vi "Package.vi"   [LabVIEW 2017, in "Scripts.lvlib"]
doc: "Builds a VI package (vip) for this project for LabVIEW 2015."
uses:
  Scripts.lvlib
  Controls/LabVIEW Versions.ctl
panel:
  # "Overview: Builds a VI Package (vip) for LabVIEW versions >= 2015\nRequirements: LabVIEW 2015, VIPM Pro, VIPM API\nInstructions: Run this VI.\n\nThis VI attempts automate the building the VIP file for this add-on as much as possible. If VIPM Pro is not available, then the VIPM API will not work, and the building of the package must be done manually. This VI automates the following manual steps:\n\n1. Save the current project for LabVIEW 2015\n    a. From the Project Explorer window, select File>>Save for Previous Version... A new dialog will appear.\n    b. Select 15.0 from the drop down menu.\n    c. Click Save.... A new dialog will appear. Create a \"target\\15.0\" folder hierarchy in the root project folder (same location as the project file,    \n        .lvproj) if it does not already exist.\n    d. Click OK. All of the contents of the project will be saved to LabVIEW 2015.\n2. Copy the Help source to the target output\n    a. Start Windows Explorer.\n    b. Navigate to the \"<project root>\\src\" folder in Windows Explorer.\n    c. Copy the \"Help\" folder to the \"target\\15.0\\src\" location.\n3. Start LabVIEW 2015 and open the \"target\\15.0\\Alphabetize Cluster Elements.lvproj\" file created in Step 1. Do NOT open any file in the \"target\\15.0\" folder in any other \n    version of LabVIEW.\n4. Build all Source Distributions defined under \"Build Specifications\" tree item in the Project Explorer. A new \"target\\15.0\\builds\" folder will be \n    created with a sub-folder for each component.\n5. Expand the \"Configs\" virtual folder in the Project Explorer and double click on the \"Alphabetize Cluster Elements.vipb\" file. This will start the VIPM application.\n6. Click the \"Build\" icon near the top of the window for the Eulogy package specification. Do NOT alter any values, but ensure \"2015\" is selected at \n    the top right.\n7. Once the package is built, it will be available at \"target\\15.0\\packages\". \n\nNote, any version newer than LabVIEW 2015 can be used to run this VI and still have the package built for LabVIEW 2015, but the LabVIEW 2015 development environment must be installed.\n\nWhen this VI runs, it will automatically start LabVIEW 2015, build all of the components, start VIPM, build the package, then close both LabVIEW 2015 and VIPM. Another VI, \"Build Target.vi\" will run during this process. Do not abort or close the VI will running.\n\nThe oldest LabVIEW version possible for this add-on is LabVIEW 2015. LabVIEW 2015 introduced shortcut menu plugins, which are an integral usability component to this add-on. If the shortcut menu items are not needed, then the oldest version possible is LabVIEW 2013, which introduced custom bookmark managers. Similarly, custom bookmark managers are an integratl usability component for this add-on. All of the features and functionality are not possible with versions older than LabVIEW 2015."
types:
  T1 = typedef "Scripts.lvlib/LabVIEW Versions.ctl" = enum16{"2009", "2010", "2011", "2012", "2013", "2014", "2015", "2016", "2017", "2018"}
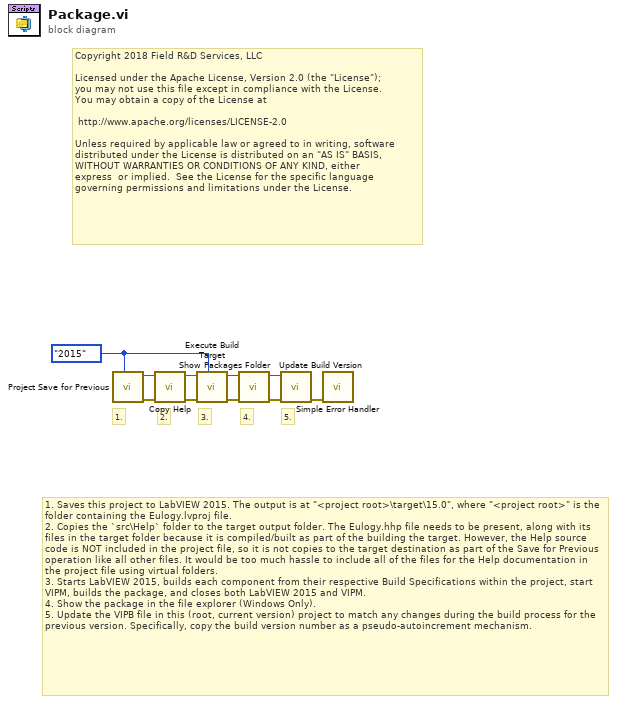
[diagram p0: block diagram]
diagram:
  w10 = LabVIEW_Versions."2015" ("LabVIEW Previous Version")
  # "5."
  # "4."
  # "3."
  # "2."
  # "Copyright 2018 Field R&D Services, LLC\n\nLicensed under the Apache License, Version 2.0 (the \"License\");\nyou may not use this file except in compliance with the License.\nYou may obtain a copy of the License at\n\n\thttp://www.apache.org/licenses/LICENSE-2.0\n\nUnless required by applicable law or agreed to in writing, software\ndistributed under the License is distributed on an \"AS IS\" BASIS,\nWITHOUT WARRANTIES OR CONDITIONS OF ANY KIND, either \nexpress  or implied.  See the License for the specific language \ngoverning permissions and limitations under the License."
  # "1. Saves this project to LabVIEW 2015. The output is at \"<project root>\\target\\15.0\", where \"<project root>\" is the folder containing the Eulogy.lvproj file.\n2. Copies the `src\\Help` folder to the target output folder. The Eulogy.hhp file needs to be present, along with its files in the target folder because it is compiled/built as part of the building the target. However, the Help source code is NOT included in the project file, so it is not copies to the target destination as part of the Save for Previous operation like all other files. It would be too much hassle to include all of the files for the Help documentation in the project file using virtual folders.\n3. Starts LabVIEW 2015, builds each component from their respective Build Specifications within the project, start VIPM, builds the package, and closes both LabVIEW 2015 and VIPM.\n4. Show the package in the file explorer (Windows Only).\n5. Update the VIPB file in this (root, current version) project to match any changes during the build process for the previous version. Specifically, copy the build version number as a pseudo-autoincrement mechanism."
  # "1."
  n1 = call "Project Save for Previous.vi"("LabVIEW Previous Version"=w10) -> ("Error Out"=w8:errorcluster, "Destination"=w6:path)  [unwired: 9 in]
  n2 = call "Copy Help.vi"("Error In"=w8, "Target Project Root In"=w6) -> ("Error Out"=w7:errorcluster, "Target Project Root Out"=w5:path)  [unwired: 8 in]
  n3 = call "Execute Build Target.vi"("LabVIEW Previous Version"=w10, "Error In"=w7, "Target Project Root In"=w5) -> ("Error Out"=w4:errorcluster, "Target Project Root Out"=w3:path)  [unwired: 7 in]
  n4 = call "Show Packages Folder.vi"("Error In"=w4, "Target Project Root In"=w3) -> ("Error Out"=w1:errorcluster, "Target Project Root Out"=w2:path)  [unwired: 8 in]
  n5 = call "Update Build Version.vi"("Error In"=w1, "Target Project Root In"=w2) -> ("Error Out"=w9:errorcluster)  [unwired: 8 in, 1 out]
  n6 = call <vilib>:"Simple Error Handler.vi"("error in (no error)"=w9) -> ()  [unwired: 4 in, 5 out]
